vi "获取数据时间段.vi"() -> (2 "end time":timestamp, 3 "start time":timestamp)   [LabVIEW 2016, in "环境动力监测库.lvlib" / "NMEA.lvlib"]
uses:
  NMEA.lvlib
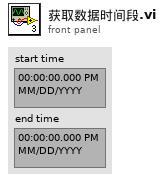
[diagram p1: front panel]
types:
  T1 = typedef "LVDateTimeRec.ctl" = cluster{"秒数的小数部分":dbl, "秒":i32, "分":i32, "时":i32, "日":i32, "月":i32, "年":i32, "天数（周）":i32, "天数（年）":i32, "DST":i32}
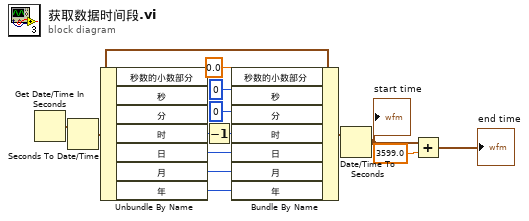
[diagram p0: block diagram]
diagram:
  n1 = Get Date/Time In Seconds() -> (seconds since 1Jan1904=w14:timestamp)
  n2 = Seconds To Date/Time(time stamp (now)=w14) -> (date time rec=w13:T1)  [unwired: 1 in]
  n3 = Unbundle By Name(w13) -> ("时"=w9:i32, "日"=w10:i32, "月"=w11:i32, "年"=w12:i32)  [unwired: 3 out]
  n4 = Decrement(x=w9) -> (x-1=w8:i32)
  n5 = Bundle By Name(cluster=w13, "秒数的小数部分"=0.0, "秒"=0, "分"=0, "时"=w8, "日"=w10, "月"=w11, "年"=w12) -> (w4:T1)
  n6 = Date/Time To Seconds(2:w4) -> (0:w3:timestamp)  [unwired: 1 in]
  "start time" <- w3
  n7 = Add(x=w3, y=3599.0) -> (x+y=→"end time":timestamp)
